vi "Noise-Circular Play.vi"(0 "Noise (in)":dbl[](array[numeric]), 2 "Init? (F)":bool, 9 "Npts":i32, 11 "error in (no error)":errorcluster) -> (4 "Noise (out)":dbl[](array[numeric]), 15 "error out":errorcluster)   [LabVIEW 2015]
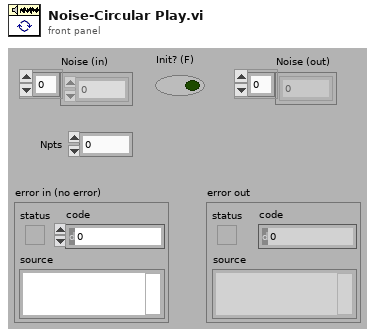
[diagram p1: front panel]
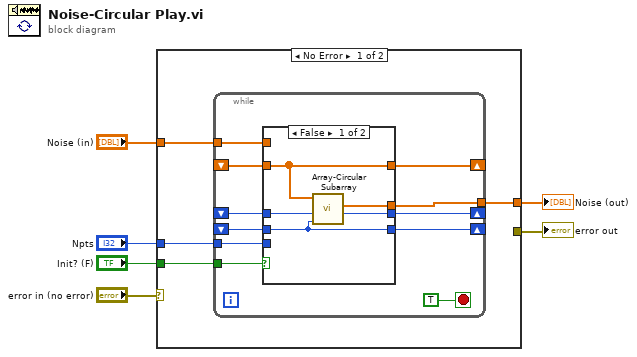
[diagram p0: block diagram]
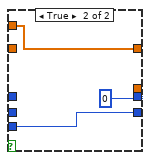
[diagram p2: hidden frame]
diagram:
  n1 = case shown="No Error" "error in (no error)" {
    selector: "error in (no error)" -> [_ w30]
    tunnel: [_ w30] -> w6
    tunnel: "Noise (in)" -> [w10 _]
    tunnel: "Init? (F)" -> [w9 _]
    tunnel: "Npts" -> [w7 _]
    tunnel: [w8 _] -> w1
    frame No Error {
      n2 = while {
        tunnel: w10 -> [w20]
        tunnel: w9 -> [w21]
        shift-right: [w19] -> _
        shift-left: _ -> [w18]
        shift-right: [w16] -> _
        shift-left: _ -> [w17]
        tunnel: [w15] -> w8
        shift-right: [w13] -> _
        shift-left: _ -> [w11]
        tunnel: w7 -> [w12]
        stop <- TRUE stop-if-true
        n3 = case shown="False" w21 {
          tunnel: w20 -> [_ w29]
          tunnel: [w26 w29] -> w19
          tunnel: w18 -> [w26 _]
          tunnel: w17 -> [w24 _]
          tunnel: [w23 0] -> w16
          tunnel: [w25 _] -> w15
          tunnel: [w22 w27] -> w13
          tunnel: w12 -> [_ w27]
          tunnel: w11 -> [w22 _]
          frame False {
            n4 = call "Array-Circular Subarray.vi"("Npts"=w22, "Offset (in)"=w24, "Array"=w26) -> ("Offset (out)"=w23:i32, "Subarray"=w25:dbl[])  [unwired: 7 in]
          }
          frame True {
          }
        }
      }
    }
    frame Error {
    }
  }
  "error out" <- w6
  "Noise (out)" <- w1
